vi "Get Channel Names.vi"(1 "Channel Settings":T1[](array[typedef])) -> (0 "Channel Names":string[](array[string]))   [LabVIEW 2021, in "Acquisition.lvlib"]
doc: "Get the Names of the channels in 'Channel Settings' (returns the names in the same order as the channels)."
uses:
  Acquisition.lvlib
  Channel Settings.ctl
  IO Device.ctl
  Sensor Type.ctl
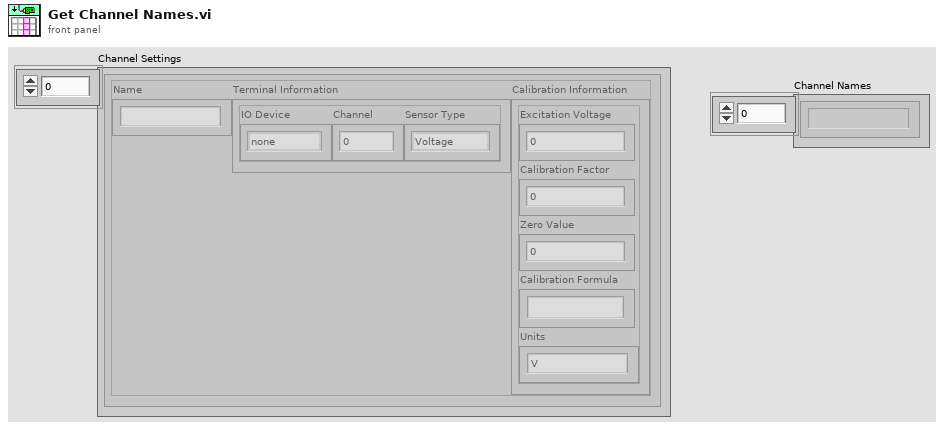
[diagram p1: front panel]
types:
  T1 = typedef "Acquisition.lvlib/Channel Settings.ctl" = cluster{"Name":string, "Terminal Information":cluster{"IO Device":T2, "Channel":i32, "Sensor Type":T3}, "Calibration Information":cluster{"Excitation Voltage":dbl, "Calibration Factor":dbl, "Zero Value":dbl, "Calibration Formula":string, "Units":string}}
  T2 = typedef "Acquisition.lvlib/IO Device.ctl" = enum16{"none", "9219", "9401"}
  T3 = typedef "Acquisition.lvlib/Sensor Type.ctl" = enum16{"Voltage", "Load", "Pressure", "Encoder"}
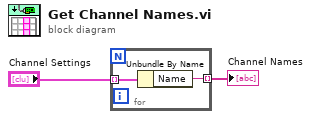
[diagram p0: block diagram]
diagram:
  n1 = for {
    tunnel: "Channel Settings" -> [w4] mode=indexing
    tunnel: [w3] -> w1 mode=indexing
    n2 = Unbundle By Name(w4) -> ("Name"=w3:string)
  }
  "Channel Names" <- w1
